vi "Disconnect All.vi"(8 "error in (no error)":errorcluster, 11 "Function in":refnum<class "Function.lvclass">) -> (0 "error out":errorcluster, 3 "Function out":refnum<class "Function.lvclass">)   [LabVIEW 2016, in "Function Actor.lvlib" / "Function.lvclass"]
uses:
  <userlib>/Common Components/Function Actor/Function.lvclass
  <userlib>/Common Components/Function Actor/Function.lvclass/Function.ctl
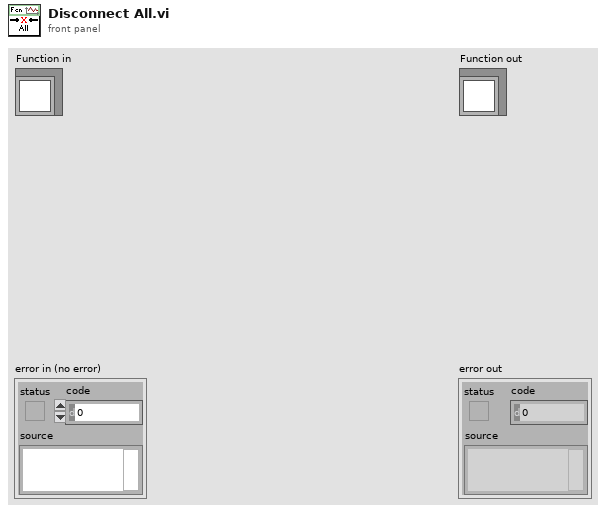
[diagram p1: front panel]
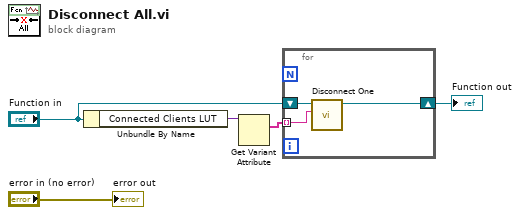
[diagram p0: block diagram]
diagram:
  n1 = Unbundle By Name("Function in") -> ("Connected Clients LUT"=w4:variant)
  n2 = Get Variant Attribute(Variant=w4) -> (names=w1:string[])  [unwired: 3 in, 3 out]
  n3 = for {
    shift-right: [w7] -> w2
    shift-left: "Function in" -> [w8]
    tunnel: w1 -> [w6] mode=indexing
    n4 = call <userlib>:"Disconnect One.vi"("GUID"=w6, "Function in"=w8) -> ("Function out"=w7:refnum<class "Function.lvclass">)  [unwired: 8 in, 1 out]
  }
  "Function out" <- w2
  "error out" <- "error in (no error)"
